vi "Read Headers.vi"(8 "error in (no error)":errorcluster, 10 "Header Names":string[](array[string]), 11 "Linked List Header in":refnum<class "Linked List Header.lvclass">) -> (0 "error out":errorcluster, 1 "Header Values":string[](array[string]), 2 "Header Names":string[](array[string]), 3 "Linked List Header out":refnum<class "Linked List Header.lvclass">, 4 "Found?":bool)   [LabVIEW 2019, in "Linked Lists.lvlib" / "Linked List Header.lvclass"]
uses:
  <vilib>/gpm_packages/@cs/linked-list/Source/Linked List/Linked List Header/Linked List Header.lvclass
  <vilib>/gpm_packages/@cs/linked-list/Source/Linked List/Linked List Header/Linked List Header.lvclass/Linked List Header.ctl
  <vilib>/gpm_packages/@cs/lookup-table/Source/LookupTable/LookupTable.lvclass/LookupTable.ctl
  e2f8eef0-0942-4649-9a12-1d946ce83b84.vi
  da017be6-abdf-4568-b31b-0faaf558a6af.vi
  <vilib>/gpm_packages/@cs/lookup-table/Source/LookupTable/Read Table Reference.vi
  e2f8eef0-0942-4649-9a12-1d946ce83b84.vi/2d273f04-058b-413c-9068-f3df89f3fd86.vi
  <vilib>/gpm_packages/@cs/lookup-table/Source/LookupTable/LookupTable.lvclass
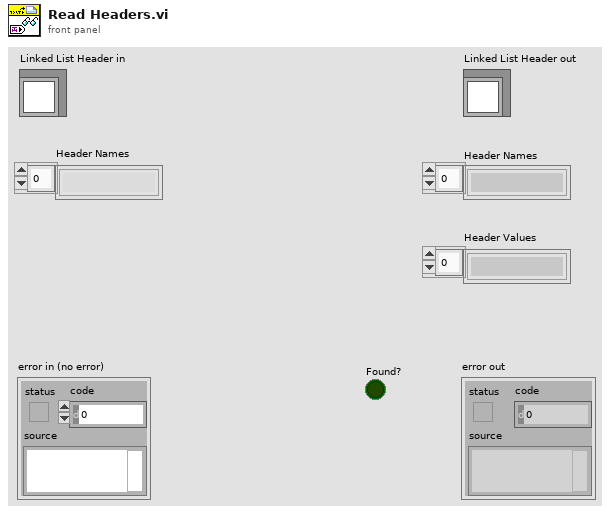
[diagram p1: front panel]
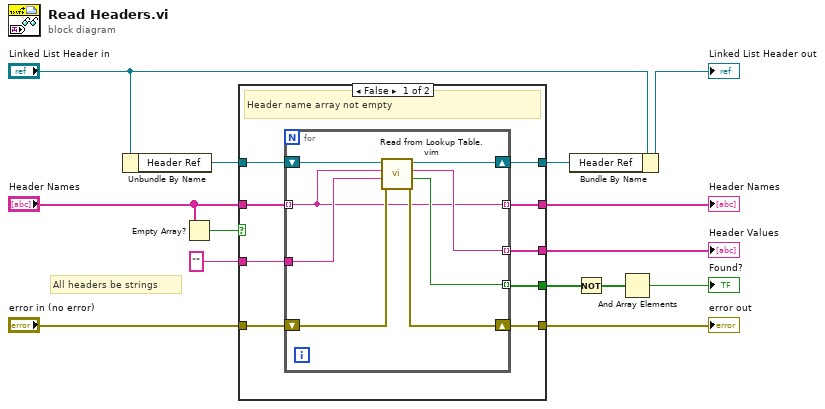
[diagram p0: block diagram]
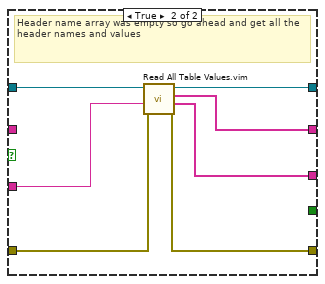
[diagram p2: hidden frame]
diagram:
  # "All headers be strings"
  n1 = Unbundle By Name("Linked List Header in") -> ("Header Ref"=w14:refnum<data-value>)
  n2 = Empty Array?(array="Header Names") -> (empty?=w2:bool)
  n3 = case shown="False" w2 {
    tunnel: w14 -> [w23 w38]
    tunnel: "error in (no error)" -> [w22 w36]
    tunnel: [w21 w35] -> w12
    tunnel: "" -> [w20 w34]
    tunnel: [w19 w37] -> w10
    tunnel: [w18 w33] -> w7
    tunnel: [w17 _] -> w6
    tunnel: "Header Names" -> [w16 _]
    tunnel: [w15 w32] -> w1
    frame False {
      # "Header name array not empty"
      n4 = for {
        shift-right: [w29] -> w21
        shift-left: w22 -> [w30]
        tunnel: w16 -> [w24] mode=indexing
        tunnel: w20 -> [w28]
        shift-right: [w27] -> w19
        shift-left: w23 -> [w31]
        tunnel: [w26] -> w18 mode=indexing
        tunnel: [w25] -> w17 mode=indexing
        tunnel: [w24] -> w15 mode=indexing
        n5 = call "Read from Lookup Table.vim"("error in (no error)"=w30, "Type"=w28, "Item Name"=w24, "LookupTable Reference"=w31) -> ("error out"=w29:errorcluster, "Not Found?"=w25:bool, "Value"=w26:string, "LookupTable Reference Out"=w27:refnum<data-value>)  [unwired: 4 in]
      }
    }
    frame True {
      # "Header name array was empty so go ahead and get all the header names and values"
      n6 = call "Read All Table Values.vim"("error in (no error)"=w36, "Type (All)"=w34, "LookupTable Reference"=w38) -> ("error out"=w35:errorcluster, "Values"=w33:string[], "Names"=w32:string[], "LookupTable Reference Out"=w37:refnum<data-value>)  [unwired: 5 in]
    }
  }
  "error out" <- w12
  "Header Values" <- w7
  "Header Names" <- w1
  n7 = Bundle By Name(cluster="Linked List Header in", "Header Ref"=w10) -> (→"Linked List Header out":refnum<class "Linked List Header.lvclass">)
  n8 = Not(x=w6) -> (.not. x?=w5:bool[])
  n9 = And Array Elements(Boolean array=w5) -> (logical AND=→"Found?":bool)
